vi "initializeDefaultStyle.vi"(8 "error in (no error)":errorcluster, 11 "MS-Excel in":refnum<class "MS-Excel.lvclass">) -> (0 "error out":errorcluster, 3 "MS-Excel out":refnum<class "MS-Excel.lvclass">)   [LabVIEW 2017, in "LabVIEW NPOI.lvlib" / "MS-Excel.lvclass"]
uses:
  MS-Excel.lvclass
  C:/Users/Neo/Desktop/Dev_Tools_BR/LabVIEW_NPOI/src/LabVIEW NPOI/Document/Document.lvclass
  Styles/Style/Style.lvclass
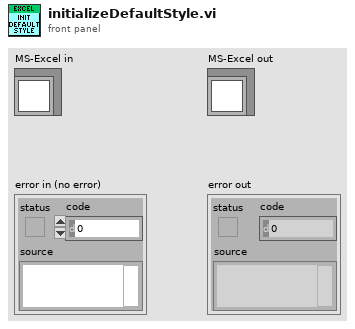
[diagram p1: front panel]
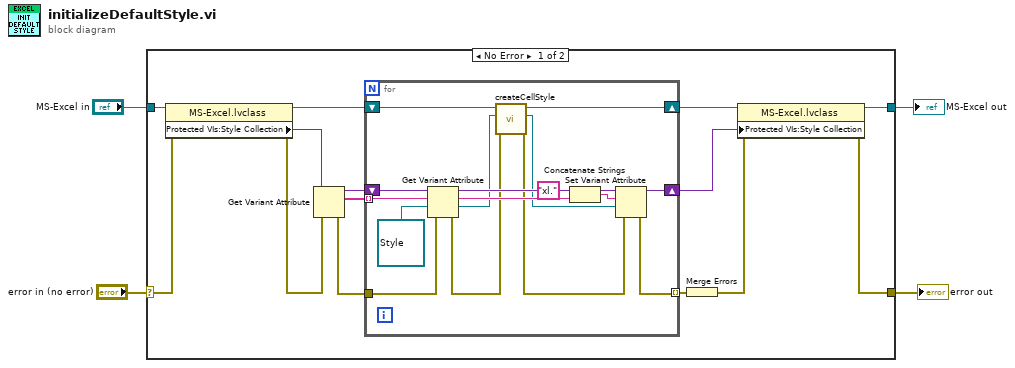
[diagram p0: block diagram]
diagram:
  n1 = case shown="No Error" "error in (no error)" {
    selector: "error in (no error)" -> [w15 w35]
    tunnel: [w7 w35] -> w3
    tunnel: [w9 w34] -> w1
    tunnel: "MS-Excel in" -> [w18 w34]
    frame No Error {
      n2 = property class="MS-Excel.lvclass"(reference=w18, error in=w15) -> (reference out=w16:refnum<class "MS-Excel.lvclass">, error out=w10:errorcluster, "Protected VIs:Style Collection"=w14:variant)
      n3 = Get Variant Attribute(Variant=w14, error in=w10) -> (duplicate Variant=w11:variant, names=w12:string[], error out=w13:errorcluster)  [unwired: 2 in, 1 out]
      n4 = for {
        shift-right: [w33] -> w17
        shift-left: w16 -> [w32]
        tunnel: w13 -> [w31]
        tunnel: w12 -> [w26] mode=indexing
        shift-right: [w27] -> w5
        shift-left: w11 -> [w30]
        tunnel: [w21] -> w8 mode=indexing
        n5 = Get Variant Attribute(Variant=w30, name=w26, default value (empty Variant)=refnum<class "Style.lvclass"> refnum ("Style out"), error in=w31) -> (duplicate Variant=w28:variant, value=w25:refnum<class "Style.lvclass">, error out=w23:errorcluster)  [unwired: 1 out]
        n6 = call-dynamic "createCellStyle.vi"("error in (no error)"=w23, "Style"=w25, "MS-Excel in"=w32) -> ("error out"=w22:errorcluster, "Cell Style"=w24:refnum<k24>, "MS-Excel out"=w33:refnum<class "MS-Excel.lvclass">)  [unwired: 6 in]
        n7 = Concatenate Strings("xl." ("string"), w26) -> (w20:string)
        n8 = Set Variant Attribute(Variant=w28, name=w20, value=w24, error in=w22) -> (Variant out=w27:variant, error out=w21:errorcluster)  [unwired: 1 out]
      }
      n9 = Merge Errors(w8) -> (w6:errorcluster)
      n10 = property class="MS-Excel.lvclass"(reference=w17, error in=w6, "Protected VIs:Style Collection"=w5) -> (reference out=w9:refnum<class "MS-Excel.lvclass">, error out=w7:errorcluster)
    }
    frame Error {
    }
  }
  "error out" <- w3
  "MS-Excel out" <- w1
